vi "Host_DDS_calc_FPGA_params.vi"(5 "Accumulator Size (bit)":i32=32, 7 "Loop Rate (Hz)":dbl, 9 "Signal Amplitude (V)":dbl=1.0, 11 "DDS Signal Frequency (Hz)":dbl=20000.0) -> (1 "AO Amplitude":u16, 2 "Phase Shift":u32, 3 "Accumulator Increment":u32, 4 "freq_adjusted?":dbl format="%#_16g")   [LabVIEW 2017]
panel:
  out "x/y":dbl
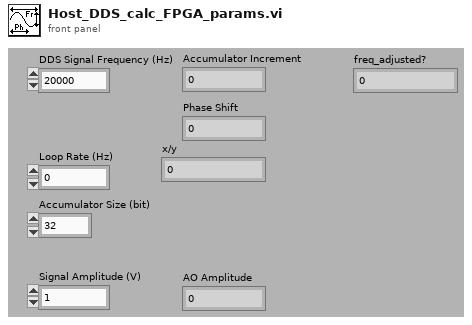
[diagram p1: front panel]
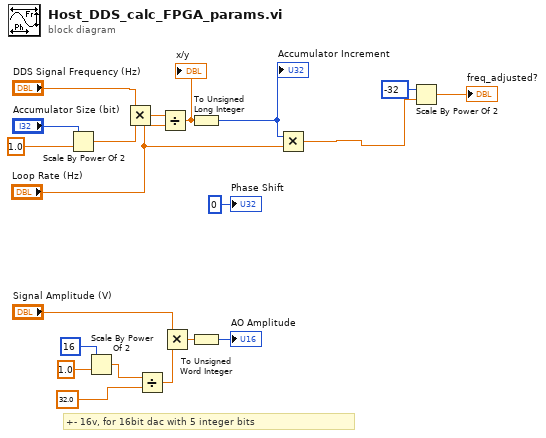
[diagram p0: block diagram]
diagram:
  # "+- 16v, for 16bit dac with 5 integer bits"
  n1 = Scale By Power Of 2(n="Accumulator Size (bit)", x=1.0) -> (x*2^n=w16:dbl)
  n2 = Scale By Power Of 2(n=i16 16, x=1.0) -> (x*2^n=w11:dbl)
  n3 = Multiply(x="DDS Signal Frequency (Hz)", y=w16) -> (x*y=w17:dbl)
  n4 = Divide(x=w11, y=32.0) -> (x/y=w13:dbl)
  n5 = Divide(x=w17, y="Loop Rate (Hz)") -> (x/y=w20:dbl)
  "x/y" <- w20
  n6 = Multiply(x="Signal Amplitude (V)", y=w13) -> (x*y=w15:dbl)
  n7 = To Unsigned Long Integer(number=w20) -> (unsigned 32bit integer=w6:u32)
  "Accumulator Increment" <- w6
  n8 = To Unsigned Word Integer(number=w15) -> (unsigned 16bit integer=→"AO Amplitude":u16)
  n9 = Multiply(x=w6, y="Loop Rate (Hz)") -> (x*y=w1:dbl)
  n10 = Scale By Power Of 2(n=i16 -32, x=w1) -> (x*2^n=→"freq_adjusted?":dbl)
  "Phase Shift" <- u32 0 ("Phase Shift")
